vi "Analyse.vi"(8 "error in (no error)":errorcluster, 11 "WelcomeHandler JSON in":refnum<class "WelcomeHandler JSON.lvclass">) -> (0 "error out":errorcluster, 3 "WelcomeHandler JSON out":refnum<class "WelcomeHandler JSON.lvclass">)   [LabVIEW 2020, in "wamplv.lvlib" / "WelcomeHandler JSON.lvclass"]
uses:
  WelcomeHandler JSON.lvclass
  WelcomeHandler JSON.lvclass/WelcomeHandler JSON.ctl
  0494aabd-d4af-4e60-bc0a-149bf2d0e5cd.vi
  SerialisedMessages/JSONMessage/WampMessage JSON.lvclass
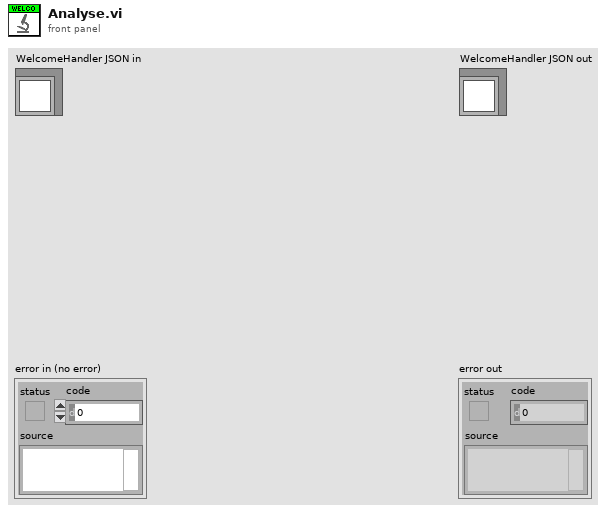
[diagram p1: front panel]
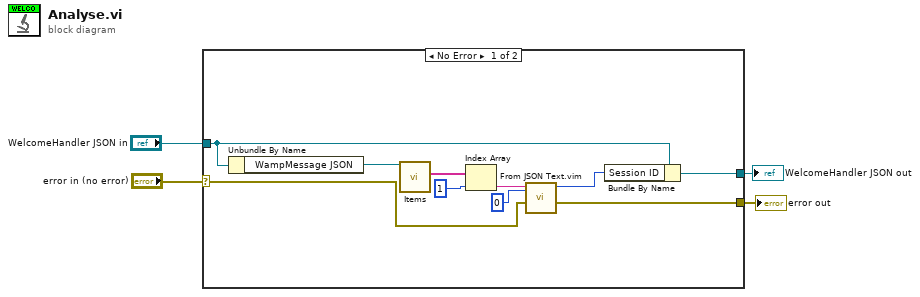
[diagram p0: block diagram]
diagram:
  n1 = case shown="No Error" "error in (no error)" {
    selector: "error in (no error)" -> [w5 w15]
    tunnel: "WelcomeHandler JSON in" -> [w6 w16]
    tunnel: [w9 w15] -> w2
    tunnel: [w8 w16] -> w1
    frame No Error {
      n2 = Unbundle By Name(w6) -> ("WampMessage JSON"=w7:refnum<class "WampMessage JSON.lvclass">)
      n3 = call-dynamic "Items.vi"("JSONMessage in"=w7) -> ("<JSON>Elements"=w13:string[])  [unwired: 9 in, 1 out]
      n4 = Index Array(array=w13, index=1) -> (element=w11:string)
      n5 = call "From JSON Text.vim"("Data Type and Default Value"=u64 0, "error in (no error)"=w5, "JSON"=w11) -> ("error out"=w9:errorcluster, "Data out"=w10:u64)  [unwired: 7 in]
      n6 = Bundle By Name(cluster=w6, "Session ID"=w10) -> (w8:refnum<class "WelcomeHandler JSON.lvclass">)
    }
    frame Error {
    }
  }
  "error out" <- w2
  "WelcomeHandler JSON out" <- w1
